vi "file saving loop.vi"(0 "files open":bool, 1 "refnums":T2, 2 "disk queues":T3, 3 "close files":bool, 4 "open files":bool, 5 "error in":errorcluster, 6 "clear":bool, 7 "data directory in":path, 8 "main vi ref":refnum<vi>) -> (13 "data directory":path, 14 "files open out":bool, 15 "refnums out":T2, 16 "time stamp (write in your lab book)":string, 17 "elements in queues":T1, 19 "error out":errorcluster)   [LabVIEW 2017]
uses:
  typedefs/queue cluster.ctl
  typedefs/reading queue.ctl
  typedefs/reading.ctl
  typedefs/readingType.ctl
  typedefs/reading1.ctl
  typedefs/refnum cluster.ctl
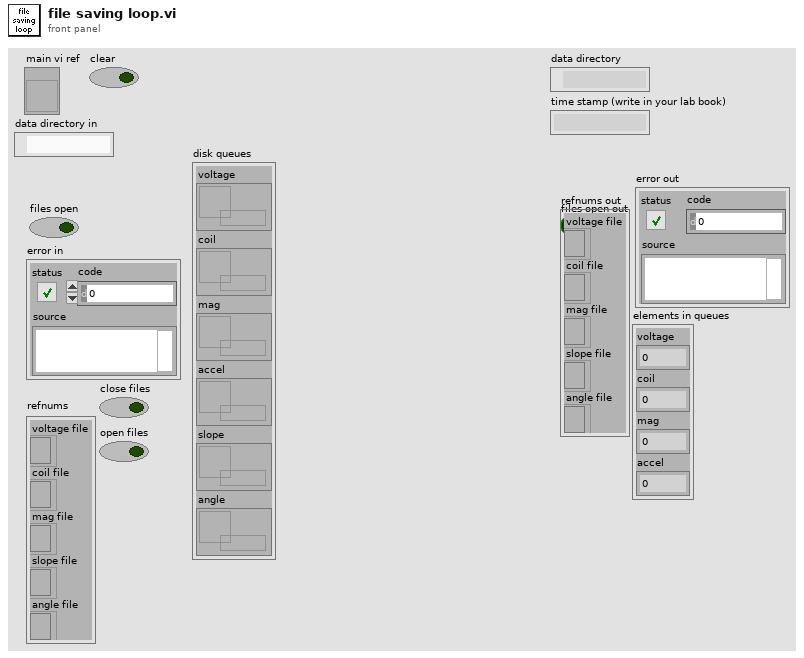
[diagram p1: front panel]
types:
  T1 = cluster{"voltage":i32, "coil":i32, "mag":i32, "accel":i32}
  T2 = typedef "refnum cluster.ctl" = cluster{"voltage file":refnum<file>, "coil file":refnum<file>, "mag file":refnum<file>, "slope file":refnum<file>, "angle file":refnum<file>}
  T3 = typedef "queue cluster.ctl" = cluster{"voltage":T4, "coil":T4, "mag":T4, "accel":T4, "slope":refnum<queue>, "angle":refnum<queue>}
  T4 = typedef "reading queue.ctl" = refnum<queue>
  T5 = cluster{"# elements in queue":i32, "# elements in queue":i32, "# elements in queue":i32, "# elements in queue":i32}
  T6 = cluster{refnum<k0>, refnum<k0>, refnum<k0>, refnum<k0>, refnum<k0>}
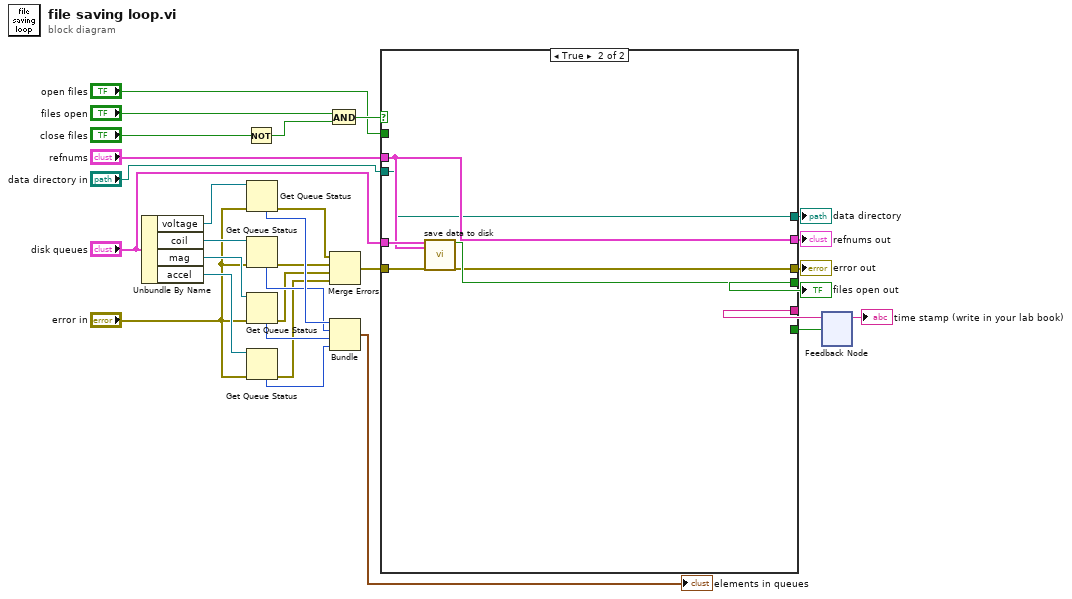
[diagram p0: block diagram]
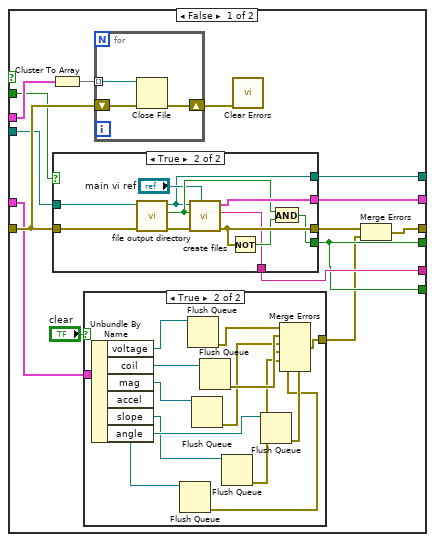
[diagram p2: hidden frame]
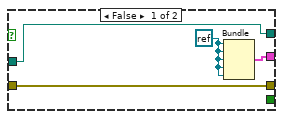
[diagram p4: hidden frame]
diagram:
  n1 = Unbundle By Name("disk queues") -> ("voltage"=w20:T4, "coil"=w19:T4, "mag"=w18:T4, "accel"=w17:T4)
  n2 = Not(x="close files") -> (.not. x?=w24:bool)
  n3 = Get Queue Status(queue=w20, error in (no error)="error in") -> (error out=w8:errorcluster, # elements in queue=w15:i32)  [unwired: 1 in, 6 out]
  n4 = Get Queue Status(queue=w19, error in (no error)="error in") -> (error out=w9:errorcluster, # elements in queue=w14:i32)  [unwired: 1 in, 6 out]
  n5 = Get Queue Status(queue=w18, error in (no error)="error in") -> (error out=w10:errorcluster, # elements in queue=w13:i32)  [unwired: 1 in, 6 out]
  n6 = Get Queue Status(queue=w17, error in (no error)="error in") -> (error out=w11:errorcluster, # elements in queue=w12:i32)  [unwired: 1 in, 6 out]
  n7 = And(x="files open", y=w24) -> (x .and. y?=w25:bool)
  n8 = Merge Errors(w8, w9, w10, w11) -> (w7:errorcluster)
  n9 = Bundle("# elements in queue"=w15, "# elements in queue"=w14, "# elements in queue"=w13, "# elements in queue"=w12) -> (→"elements in queues":T5)  [unwired: 1 in]
  n10 = case shown="True" w25 {
    tunnel: w7 -> [w42 w83]
    tunnel: "disk queues" -> [w34 w82]
    tunnel: "refnums" -> [w45 w80]
    tunnel: [w35 w81] -> w27
    tunnel: [w41 w80] -> w26
    tunnel: [w32 w79] -> w21
    tunnel: "open files" -> [w39 _]
    tunnel: [w38 w78] -> w4
    tunnel: "data directory in" -> [w37 w78]
    tunnel: [w36 _] -> w3
    tunnel: [w35 _] -> w2
    frame False {
      n11 = Cluster To Array(cluster=w45) -> (array=w44:refnum<file>[])
      n12 = case shown="True" w39 {
        tunnel: w42 -> [w62 w71]
        tunnel: [w63 w74] -> w41
        tunnel: [w62 w73] -> w40
        tunnel: [_ w69] -> w35
        tunnel: [w60 w66] -> w38
        tunnel: w37 -> [w60 w65]
        tunnel: [_ w64] -> w36
        frame False {
          w61 = refnum<k0> refnum
          n13 = Bundle(w61, w61, w61, w61, w61) -> (w63:T6)  [unwired: 1 in]
        }
        frame True {
          n14 = call "file output directory.vi"("error in"=w71, "data directory in"=w65) -> ("error out"=w70:errorcluster, "exists"=w68:bool, "data directory"=w66:path)  [unwired: 7 in]
          n15 = call "create files.vi"("main vi ref"="main vi ref", "error in"=w70, "create files"=w68, "base path"=w66) -> ("error out"=w73:errorcluster, "date/time string"=w64:string, "refnums"=w74:T2)  [unwired: 5 in]
          n16 = Not(x=w73) -> (.not. x?=w72:bool)
          n17 = And(x=w68, y=w72) -> (x .and. y?=w69:bool)
        }
      }
      n18 = case shown="True" "clear" {
        tunnel: w34 -> [_ w59]
        tunnel: [_ w50] -> w31
        frame False {
        }
        frame True {
          n19 = Unbundle By Name(w59) -> ("voltage"=w58:T4, "coil"=w57:T4, "mag"=w56:T4, "accel"=w55:T4, "slope"=w49:refnum<queue>, "angle"=w48:refnum<queue>)
          n20 = Flush Queue(queue=w48) -> (error out=w46:errorcluster)  [unwired: 1 in, 2 out]
          n21 = Flush Queue(queue=w58) -> (error out=w54:errorcluster)  [unwired: 1 in, 2 out]
          n22 = Flush Queue(queue=w56) -> (error out=w52:errorcluster)  [unwired: 1 in, 2 out]
          n23 = Flush Queue(queue=w57) -> (error out=w53:errorcluster)  [unwired: 1 in, 2 out]
          n24 = Flush Queue(queue=w49) -> (error out=w47:errorcluster)  [unwired: 1 in, 2 out]
          n25 = Flush Queue(queue=w55) -> (error out=w51:errorcluster)  [unwired: 1 in, 2 out]
          n26 = Merge Errors(w54, w53, w52, w51, w47, w46) -> (w50:errorcluster)
        }
      }
      n27 = for {
        tunnel: w44 -> [w75] mode=indexing
        shift-right: [w76] -> w43
        shift-left: w42 -> [w77]
        n28 = Close File(refnum=w75, error in=w77) -> (error out=w76:errorcluster)  [unwired: 1 out]
      }
      n29 = call <vilib>:"Clear Errors.vi"("error in (no error)"=w43) -> ()  [unwired: 5 in, 2 out]
      n30 = Merge Errors(w40, w31) -> (w32:errorcluster)
    }
    frame True {
      n31 = call "save data to disk.vi"("disk queues"=w82, "refnums"=w80, "error in"=w83) -> ("files open"=w81:bool, "error out"=w79:errorcluster)  [unwired: 15 in]
    }
  }
  "files open out" <- w27
  "refnums out" <- w26
  "error out" <- w21
  "data directory" <- w4
  n32 = feedback-in #1(w3, w2) -> ()
  n33 = feedback #1() -> (→"time stamp (write in your lab book)":string)  [unwired: 1 in]
